vi "Maps-Set API Key.vi"(0 "Google Maps Resource Out in":T1, 7 "Google Maps API Key":string, 11 "error in (no error)":errorcluster) -> (4 "Google Maps Resource Out out":T1, 15 "error out":errorcluster)   [LabVIEW 2020]
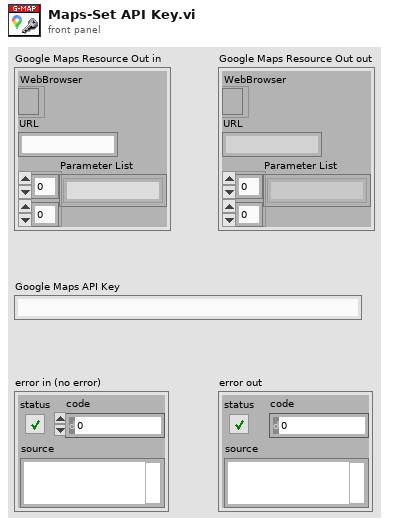
[diagram p1: front panel]
types:
  T1 = cluster{"WebBrowser":refnum<k7>, "URL":string, "Parameter List":string[][]}
  T2 = cluster{"Key":string, "Google Maps API Key":string}
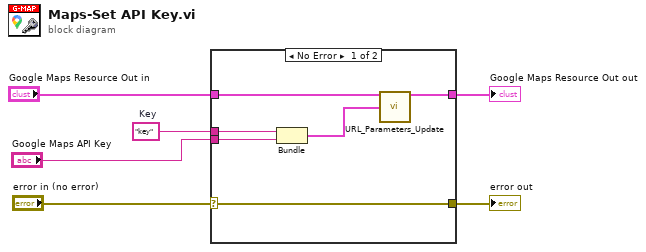
[diagram p0: block diagram]
diagram:
  w4 = "key"  # Key
  n1 = case shown="No Error" "error in (no error)" {
    selector: "error in (no error)" -> [w12 w14]
    tunnel: "Google Maps Resource Out in" -> [w11 w13]
    tunnel: "Google Maps API Key" -> [w8 _]
    tunnel: [w12 w14] -> w6
    tunnel: [w10 w13] -> w5
    tunnel: w4 -> [w9 _]
    frame No Error {
      n2 = Bundle("Key"=w9, "Google Maps API Key"=w8) -> (w7:T2)  [unwired: 1 in]
      n3 = call "URL_Parameters_Update.vi"("Google Maps Resource In"=w11, "URL Parameter"=w7) -> ("Google Maps Resource Out"=w10:T1)  [unwired: 13 in]
    }
    frame Error {
    }
  }
  "error out" <- w6
  "Google Maps Resource Out out" <- w5
